vi "SETREFdll.vi"(8 "error in (no error)":errorcluster, 11 "Inputs":T2) -> (0 "error out":errorcluster, 3 "Outputs":T1)   [LabVIEW 2016]
doc: "subroutine SETREFdll(hrf, ixflag, x0, h0, s0, t0, p0, ierr, herr, hrf_length, herr_length)\n\nSet reference state enthalpy and entropy.\n\nThis subroutine must be called after SETUP; it need not be called at all if the reference state specified in the call\nto SETUP is to be used.\n\nINPUTS:\nhrf -- Reference state for thermodynamic calculations (character*3) \n ‘NBP’: h,s = 0 at normal boiling point(s) \n ‘ASH’: h,s = 0 for saturated liquid at -40 C (ASHRAE convention) \n ‘IIR’: h = 200 kJ/kg, s = 1 kJ/kg-K for sat. liquid at 0 C (IIR convention) \n ‘DEF’: default reference state as specified in fluid file \n ‘OTH’: other, as specified by h0, s0, T0, P0 (real gas state) ‘OT0’: other, as specified by h0, s0, T0, P0 (ideal-gas state) \n ‘NA’ : not applicable, do not set up reference state (for use in debugging or fitting) \n ‘???’: set hrf to the value of the current reference state and exit\nixflag -- Composition flag: 1 - Reference state applied to pure components \n 2 - Reference state applied to mixture x0 \n\nThe following input has meaning only if ixflag = 2:\nx0 -- Composition for which h0 and s0 apply; array(1:nc) (array of mole fractions) \n This is useful for mixtures of a predefined composition, \n e.g., refrigerant blends such as R410A. \n\nThe following inputs have meaning only if hrf = ‘OTH’ or ‘OT0’:\nh0 -- Reference state enthalpy at T0, P0, and x0 [J/mol]\ns0 -- Reference state entropy at T0, P0, and x0 [J/mol-K]\nt0 -- Reference state temperature [K] T0 = -1 indicates saturated liquid at normal boiling point (bubble point for a mixture)\np0 -- Reference state pressure [kPa] P0 = -1 indicates saturated liquid at T0 (and x0) P0 = -2 indicates saturated vapor at T0 \n (and x0)\n\nOUTPUTS:\nierr -- Error flag: 0 - Successful \n 22 - Tmin > Tref for IIR reference state \n 23 - Tcrit < Tref for IIR reference state \n 24 - Tmin > Tref for ASHRAE reference state\n 25 - Tcrit < Tref for ASHRAE reference state \n 26 - Tmin > Tnbp for NBP reference state \n 27 - Tref, Pref for OTH reference state outside limits \n -28 - Can’t apply ‘DEF’ to mixture; will apply to pure components \n -29 - Unknown reference state specified; will use ‘DEF’ \n 119 - Convergence failure in calculating reference state\nherr -- Error string (character*255)\nhrf_length -- length of variable hrf (default: 3)\nherr_length -- length of variable herr (default: 255)"
uses:
  REFPROP.DLL
panel:
  # "REFPROP-SETREFdll.vi"
  # "void  SETREFdll(CStr hrf, int32_t *ixflag, double *x0, double *h0, double *s0, double *t0, double *p0, int32_t *ierr, CStr herr, int32_t hrf_length, int32_t herr_length)"
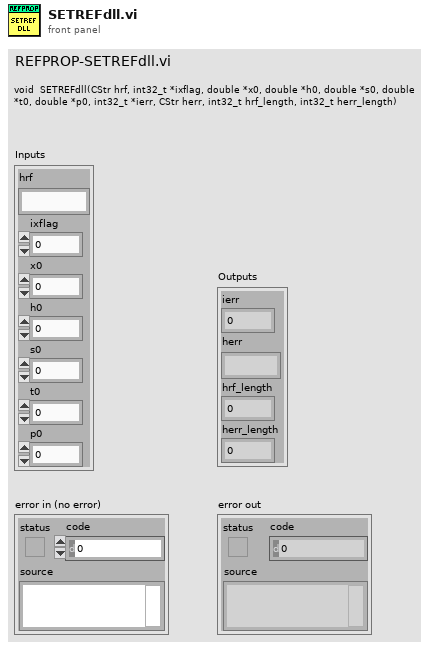
[diagram p1: front panel]
types:
  T1 = cluster{"ierr":i32, "herr":string, "hrf_length":i32, "herr_length":i32}
  T2 = cluster{"hrf":string, "ixflag":i32, "x0":dbl, "h0":dbl, "s0":dbl, "t0":dbl, "p0":dbl}
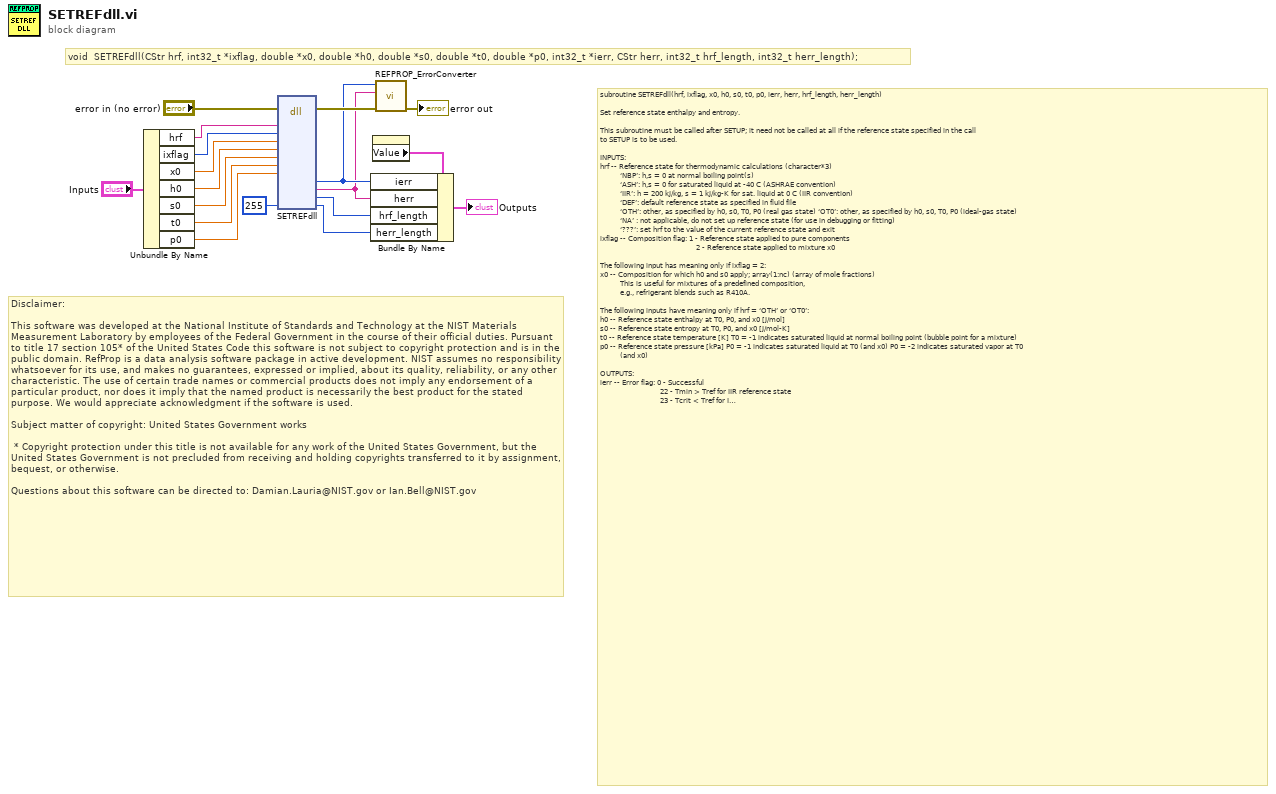
[diagram p0: block diagram]
diagram:
  # "Disclaimer:\n\nThis software was developed at the National Institute of Standards and Technology at the NIST Materials Measurement Laboratory by employees of the Federal Government in the course of their official duties. Pursuant to title 17 section 105* of the United States Code this software is not subject to copyright protection and is in the public domain. RefProp is a data analysis software package in active development. NIST assumes no responsibility whatsoever for its use, and makes no guarantees, expressed or implied, about its quality, reliability, or any other characteristic. The use of certain trade names or commercial products does not imply any endorsement of a particular product, nor does it imply that the named product is necessarily the best product for the stated purpose. We would appreciate acknowledgment if the software is used.\n \nSubject matter of copyright: United States Government works\n  \n * Copyright protection under this title is not available for any work of the United States Government, but the United States Government is not precluded from receiving and holding copyrights transferred to it by assignment, bequest, or otherwise.\n\nQuestions about this software can be directed to: Damian.Lauria@NIST.gov or Ian.Bell@NIST.gov"
  # "void  SETREFdll(CStr hrf, int32_t *ixflag, double *x0, double *h0, double *s0, double *t0, double *p0, int32_t *ierr, CStr herr, int32_t hrf_length, int32_t herr_length);"
  # "subroutine SETREFdll(hrf, ixflag, x0, h0, s0, t0, p0, ierr, herr, hrf_length, herr_length)\n\nSet reference state enthalpy and entropy.\n\nThis subroutine must be called after SETUP; it need not be called at all if the reference state specified in the call\nto SETUP is to be used.\n\nINPUTS:\nhrf -- Reference state for thermodynamic calculations (character*3) \n          ‘NBP’: h,s = 0 at normal boiling point(s) \n          ‘ASH’: h,s = 0 for saturated liquid at -40 C (ASHRAE convention) \n          ‘IIR’: h = 200 kJ/kg, s = 1 kJ/kg-K for sat. liquid at 0 C (IIR convention) \n          ‘DEF’: default reference state as specified in fluid file \n          ‘OTH’: other, as specified by h0, s0, T0, P0 (real gas state) ‘OT0’: other, as specified by h0, s0, T0, P0 (ideal-gas state) \n          ‘NA’ : not applicable, do not set up reference state (for use in debugging or fitting) \n          ‘???’: set hrf to the value of the current reference state and exit\nixflag -- Composition flag: 1 - Reference state applied to pure components \n                                                2 - Reference state applied to mixture x0 \n\nThe following input has meaning only if ixflag = 2:\nx0 -- Composition for which h0 and s0 apply; array(1:nc) (array of mole fractions) \n          This is useful for mixtures of a predefined composition, \n          e.g., refrigerant blends such as R410A. \n\nThe following inputs have meaning only if hrf = ‘OTH’ or ‘OT0’:\nh0 -- Reference state enthalpy at T0, P0, and x0 [J/mol]\ns0 -- Reference state entropy at T0, P0, and x0 [J/mol-K]\nt0 -- Reference state temperature [K] T0 = -1 indicates saturated liquid at normal boiling point (bubble point for a mixture)\np0 -- Reference state pressure [kPa] P0 = -1 indicates saturated liquid at T0 (and x0) P0 = -2 indicates saturated vapor at T0  \n          (and x0)\n\nOUTPUTS:\nierr -- Error flag: 0 - Successful \n                              22 - Tmin > Tref for IIR reference state \n                              23 - Tcrit < Tref for IIR reference state \n                              24 - Tmin > Tref for ASHRAE reference state\n                              25 - Tcrit < Tref for ASHRAE reference state \n                              26 - Tmin > Tnbp for NBP reference state \n                              27 - Tref, Pref for OTH reference state outside limits \n                            -28 - Can’t apply ‘DEF’ to mixture; will apply to pure components \n                            -29 - Unknown reference state specified; will use ‘DEF’ \n                              119 - Convergence failure in calculating reference state\nherr -- Error string (character*255)\nhrf_length -- length of variable hrf (default: 3)\nherr_length -- length of variable herr (default: 255)"
  n1 = Unbundle By Name("Inputs") -> ("hrf"=w13:string, "ixflag"=w12:i32, "x0"=w11:dbl, "h0"=w10:dbl, "s0"=w9:dbl, "t0"=w8:dbl, "p0"=w7:dbl)
  n2 = dll-call lib="S:/009 - Testing/02 - Performance Testing/REFPROP/REFPROP.*" fn="SETREFdll"(error in="error in (no error)", "hrf"=w13, "ixflag"=w12, "x0"=w11, "h0"=w10, "s0"=w9, "t0"=w8, "p0"=w7, "herr_length"=255 ("ln2")) -> (error out=w17:errorcluster, "ierr"=w2:i32, "herr"=w1:string, "hrf_length"=w5:i32, "herr_length"=w4:i32)  [unwired: 13 in, 1 out]
  n3 = property on="Outputs" class="Clust (strict)"() -> ("Value"=w6:T1)  [unwired: 2 in, 2 out]
  n4 = Bundle By Name(cluster=w6, "ierr"=w2, "herr"=w1, "hrf_length"=w5, "herr_length"=w4) -> (→"Outputs":T1)
  n5 = call "REFPROP_ErrorConverter.vi"("error in (no error)"=w17, "Error Message"=w1, "Error Code"=w2) -> ("error out"=→"error out":errorcluster)  [unwired: 8 in]
